vi "Generate Fourier Vector.vi"(11 "degree":u16) -> (3 "Fourier Matrix":cdb[](array[numeric]))   [LabVIEW 2025]
uses:
  <vilib>/Analysis/Matrix/Numeric/Conversions/Array To Matrix - CA2.vi
  <vilib>/Analysis/Matrix/Numeric/Conversions/Matrix To Array - CM.vi
  <vilib>/Analysis/Matrix/NI_Matrix.lvlib
panel:
  in  "override":bool
  out "Array":cdb[][](array[numeric])
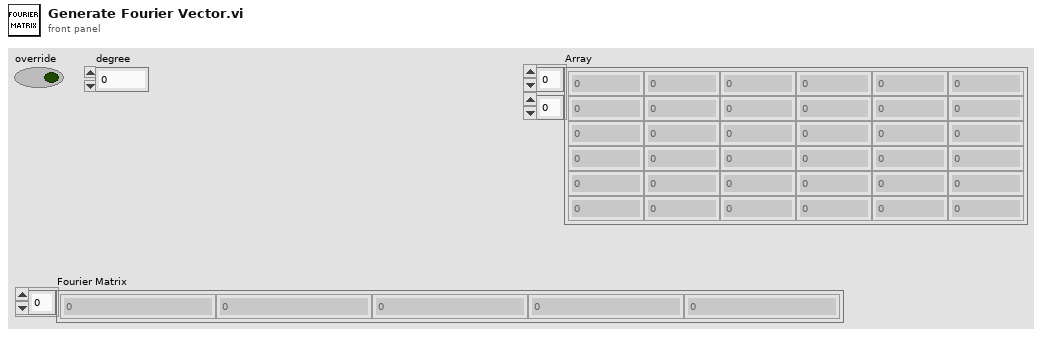
[diagram p1: front panel]
types:
  T1 = typedef "NI_Matrix.lvlib/ComplexMatrix.ctl" = cdb[][]
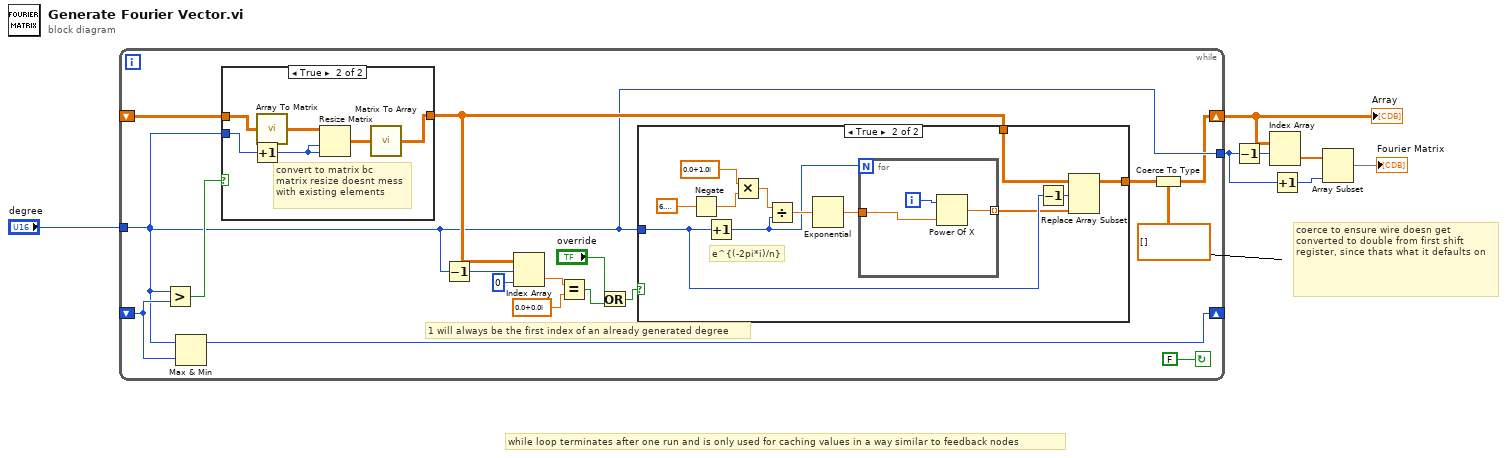
[diagram p0: block diagram]
diagram:
  # "coerce to ensure wire doesn get converted to double from first shift register, since thats what it defaults on"
  # "while loop terminates after one run and is only used for caching values in a way similar to feedback nodes"
  n1 = while {
    tunnel: "degree" -> [w15]
    shift-right: [w22] -> _
    shift-left: _ -> [w23]
    shift-right: [w9] -> w6
    shift-left: _ -> [w20]
    tunnel: [w15] -> w2
    stop <- FALSE continue-if-true
    # "1 will always be the first index of an already generated degree"
    n2 = Greater?(x=w15, y=w23) -> (0:w21:bool)
    n3 = Max & Min(x=w15, y=w23) -> (max(x,y)=w22:u16)  [unwired: 1 out]
    n4 = case shown="True" w21 {
      tunnel: w20 -> [w25 w30]
      tunnel: w15 -> [_ w27]
      tunnel: [w25 w28] -> w16
      frame False {
      }
      frame True {
        # "convert to matrix bc \nmatrix resize doesnt mess\nwith existing elements"
        n5 = Increment(x=w27) -> (x+1=w26:u16)
        n6 = call-poly <vilib>:"Array To Matrix.vi"("Complex 2D Array"=w30) -> ("Complex Matrix"=w31:T1)
        n7 = Resize Matrix(1:w26, 2:w26, 4:w31) -> (0:w29:T1)
        n8 = call-poly <vilib>:"Matrix To Array.vi"("Complex Matrix"=w29) -> ("Complex 2D Array"=w28:cdb[][])
      }
    }
    n9 = Decrement(x=w15) -> (x-1=w14:u16)
    n10 = Index Array(array=w16, index (row)=w14, index (col)=0 ("disabled index (col)")) -> (element=w18:cdb)
    n11 = Equal?(x=w18, y=cdb 0.0+0.0i) -> (x = y?=w11:bool)
    n12 = Or(x="override", y=w11) -> (x .or. y?=w13:bool)
    n13 = case shown="True" w13 {
      tunnel: w15 -> [_ w35]
      tunnel: w16 -> [w32 w38]
      tunnel: [w32 w37] -> w10
      frame False {
      }
      frame True {
        # "e^{(-2pi*i)/n}"
        n14 = Negate(x=6.283185307179586) -> (-x=w43:dbl)
        n15 = Increment(x=w35) -> (x+1=w36:u16)
        n16 = Multiply(x=cdb 0.0+1.0i ("x + iy"), y=w43) -> (x*y=w42:cdb)
        n17 = Divide(x=w42, y=w36) -> (x/y=w44:cdb)
        n18 = Exponential(1:w44) -> (0:w40:cdb)
        n19 = for {
          N: w36 -> [_]
          tunnel: w40 -> [w47]
          tunnel: [w46] -> w33 mode=indexing
          i -> [w45]
          n20 = Power Of X(1:w47, 2:w45) -> (0:w46:cdb)
        }
        n21 = Decrement(x=w35) -> (x-1=w34:u16)
        n22 = Replace Array Subset(array=w38, new element=w33, index (row)=w34) -> (w37:cdb[][])  [unwired: 1 in]
      }
    }
    n23 = Coerce To Type(0:w10, 1:cdb[][] [] ("Array")) -> (2:w9:cdb[][])
  }
  "Array" <- w6
  n24 = Decrement(x=w2) -> (x-1=w5:u16)
  n25 = Index Array(array=w6, index (row)=w5) -> (element=w4:cdb[])  [unwired: 1 in]
  n26 = Increment(x=w2) -> (x+1=w1:u16)
  n27 = Array Subset(array=w4, length=w1) -> (→"Fourier Matrix":cdb[])  [unwired: 1 in]
